vi "GD_GesamtKonz_Teil_back_calc.vi"(4 "Einheiten":string[](array[string]), 5 "ohne Einheiten":bool, 6 "Konzentration der Komponenten":dbl[](array[numeric]), 7 "Stufen":string, 9 "Gesamtkonzentration":dbl, 10 "Zeile":i32, 11 "Stufen Tabellen in (Eingang)":string[][][](array[string])) -> (3 "Stufen Tabellen in (Ausgang)":string[][][](array[string]))   [LabVIEW 2020, in "Linearisierung v2.lvlib" / "Gasteiler.lvlib"]
uses:
  Gasteiler.lvlib
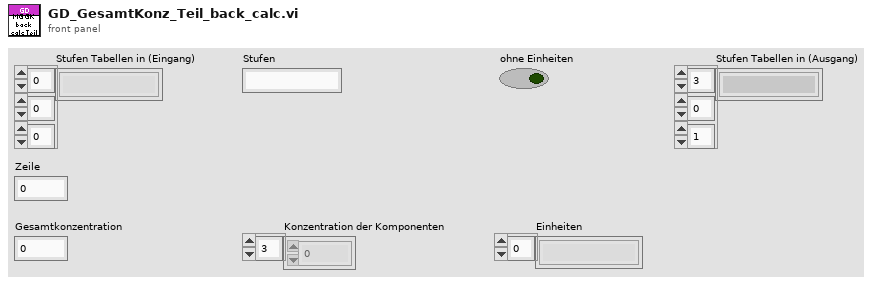
[diagram p1: front panel]
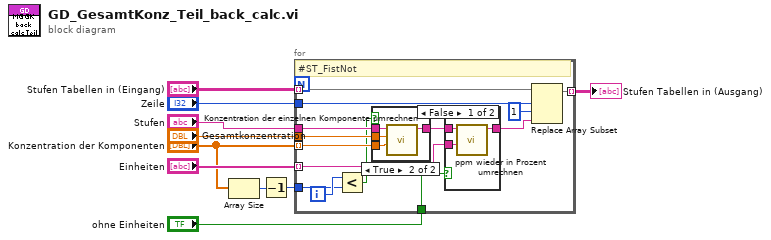
[diagram p0: block diagram]
diagram:
  n1 = Array Size(array="Konzentration der Komponenten") -> (size(s)=w3:i32)
  n2 = Decrement(x=w3) -> (x-1=w1:i32)
  n3 = for {
    tunnel: "Konzentration der Komponenten" -> [w22] mode=indexing
    tunnel: "Einheiten" -> [w21] mode=indexing
    tunnel: "Stufen" -> [w23]
    tunnel: "Gesamtkonzentration" -> [w20]
    tunnel: "Zeile" -> [w17]
    tunnel: "Stufen Tabellen in (Eingang)" -> [w16] mode=indexing
    tunnel: [w15] -> w10 mode=indexing
    tunnel: "ohne Einheiten" -> [w14]
    tunnel: w1 -> [w12]
    i -> [w13]
    # "#ST_FistNot"
    n4 = Less?(x=w13, y=w12) -> (x < y?=w11:bool)
    n5 = case shown="True" w11 {
      tunnel: [w25 w29] -> w24
      tunnel: w23 -> [w25 w28]
      tunnel: w22 -> [_ w27]
      tunnel: w20 -> [_ w26]
      frame False {
      }
      frame True {
        n6 = call "Konzentration der einzelnen Komponente umrechnen.vi"("Teilkonzentration"=w27, "Gesamtkonzentration"=w26, "Werteingang"=w28) -> ("Wertausgang"=w29:string)  [unwired: 8 in]
      }
    }
    n7 = case shown="False" w14 {
      tunnel: w24 -> [w32 w33]
      tunnel: w21 -> [w31 _]
      tunnel: [w30 w33] -> w18
      frame False {
        n8 = call "ppm wieder in Prozent umrechnen.vi"("Einheit"=w31, "Werteingang"=w32) -> ("Wertausgang"=w30:string)  [unwired: 9 in]
      }
      frame True {
      }
    }
    n9 = Replace Array Subset(array=w16, new element=w18, index (row)=w17, index (col)=1 ("Deaktivierter Index (Spalte)")) -> (w15:string[][])
  }
  "Stufen Tabellen in (Ausgang)" <- w10
